vi "Memory.Pointer.Set Address.vi"(10 "address":u64 format="%016x", 11 "Pointer in":refnum<class "Memory.Pointer.lvclass">) -> (3 "Pointer out":refnum<class "Memory.Pointer.lvclass">)   [LabVIEW 2016, in "Memory Manager.lvlib" / "Memory.Pointer.lvclass"]
uses:
  Memory.Pointer.lvclass
  Memory.Pointer.lvclass/Memory.Pointer.ctl
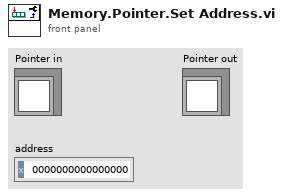
[diagram p1: front panel]
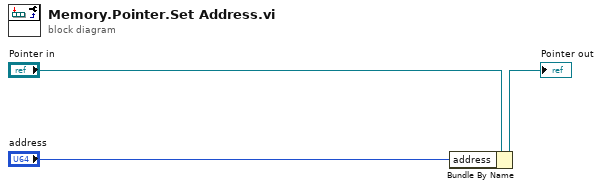
[diagram p0: block diagram]
diagram:
  n1 = Bundle By Name(cluster="Pointer in", "address"="address") -> (→"Pointer out":refnum<class "Memory.Pointer.lvclass">)
